vi "DAQ_PS Close.vi"(0 "DAQmx Task In":refnum<k21>, 11 "error in (no error)":errorcluster) -> (15 "error out":errorcluster)   [LabVIEW 2021, in "DAQ_Power Supply Source and Measure.lvlib"]
doc: "Closes and clears the power supply task."
uses:
  DAQ_Power Supply Source and Measure.lvlib
panel:
  # "Inputs"
  # "Outputs"
  # "Overview:\nThis VI closes the power supply task reference\n\nHardware Requirement: TS-15200\n\nSoftware Requirement: NI DAQmx 22Q4 or later\n\n\nInstructions:\n1. Input the power supply task through DAQmx Task In control\n2. This VI aborts and clears the Power supply DAQmx Task"
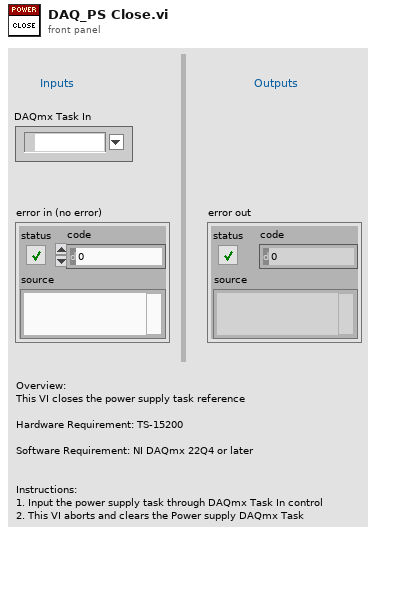
[diagram p1: front panel]
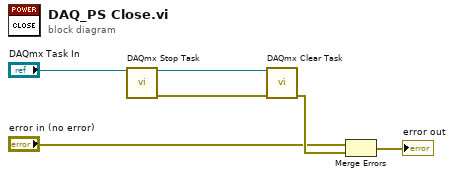
[diagram p0: block diagram]
diagram:
  n1 = call <vilib>:"DAQmx Stop Task.vi"("task/channels in"="DAQmx Task In") -> ("task out"=w6:refnum<k21>, "error out"=w5:errorcluster)  [unwired: 13 in]
  n2 = call <vilib>:"DAQmx Clear Task.vi"("task in"=w6, "error in"=w5) -> ("error out"=w4:errorcluster)  [unwired: 13 in]
  n3 = Merge Errors("error in (no error)", w4) -> (→"error out":errorcluster)
